vi "Display AppBar.vi"(8 "error in (no error)":errorcluster, 9 "AppBar Enqueuer":refnum<class "Message Enqueuer.lvclass">, 11 "MainController in":refnum<class "MainController.lvclass">) -> (0 "error out":errorcluster, 3 "MainController out":refnum<class "MainController.lvclass">)   [LabVIEW 2012, in "Win8uiFramework.lvlib" / "MainController.lvclass"]
uses:
  MainController.lvclass
  <vilib>/ActorFramework/Message Enqueuer/Message Enqueuer.lvclass
  Visibility Direction.ctl
  Visiblity States.ctl
  MainController.lvclass/MainController.ctl
  Insert Into SubPanel Msg.lvclass/Insert Into SubPanel Msg.ctl
  <vilib>/ActorFramework/Message Enqueuer/Message Enqueuer.lvclass/Message Enqueuer.ctl
  Read AppBar SubPanel.vi
  Read AppBar Enqueuer.vi
  Read AppBar State.vi
  Write AppBar Enqueuer.vi
  Write AppBar State.vi
  <vilib>/ActorFramework/Message Enqueuer/Enqueue.vi
  <vilib>/ActorFramework/Message Priority Queue/Priority Enqueue.vi
  <vilib>/Utility/error.llb/Simple Error Handler.vi
  Insert Into SubPanel Msg.lvclass
  Win8uiFramework.lvlib
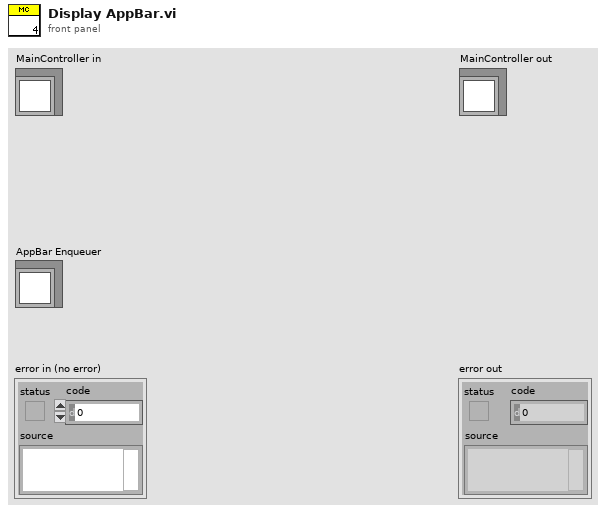
[diagram p1: front panel]
types:
  T1 = typedef "Win8uiFramework.lvlib/MainController.lvclass/Visiblity States.ctl" = enum16{"Disabled", "Hidden - Unpopulated", "Hidden - Populated", "Visible"}
  T2 = typedef "Win8uiFramework.lvlib/Visibility Direction.ctl" = enum16{"Show", "Hide"}
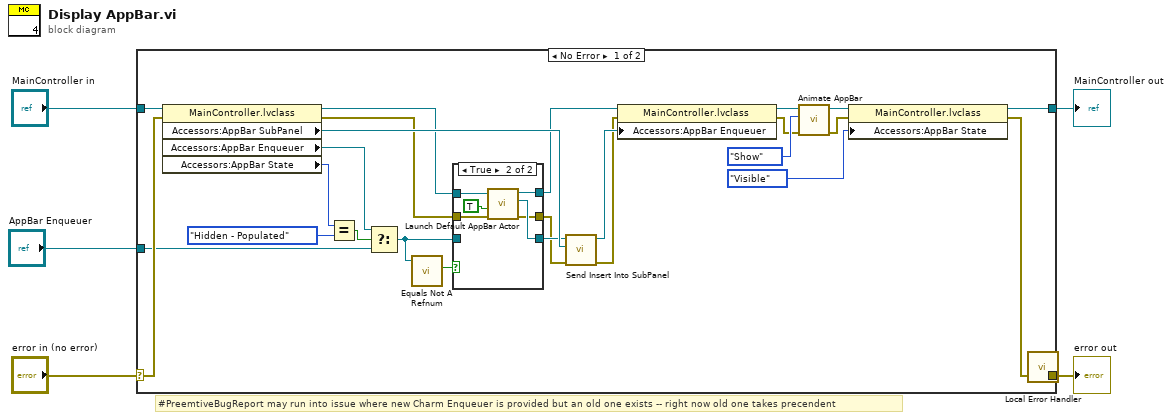
[diagram p0: block diagram]
diagram:
  # "#PreemtiveBugReport may run into issue where new Charm Enqueuer is provided but an old one exists -- right now old one takes precendent"
  n1 = case shown="No Error" "error in (no error)" {
    selector: "error in (no error)" -> [w26 w42]
    tunnel: [w6 w42] -> w4
    tunnel: [w22 w41] -> w2
    tunnel: "MainController in" -> [w31 w41]
    tunnel: "AppBar Enqueuer" -> [w18 _]
    frame No Error {
      n2 = property class="MainController.lvclass"(reference=w31, error in=w26) -> (reference out=w10:refnum<class "MainController.lvclass">, error out=w12:errorcluster, "Accessors:AppBar SubPanel"=w29:refnum<vi>, "Accessors:AppBar Enqueuer"=w15:refnum<class "Message Enqueuer.lvclass">, "Accessors:AppBar State"=w17:T1)
      n3 = Equal?(x=w17, y=Visiblity_States."Hidden - Populated") -> (x = y?=w19:bool)
      n4 = Select(t=w15, s=w19, f=w18) -> (s? t:f=w13:refnum<class "Message Enqueuer.lvclass">)
      n5 = call <vilib>:"Equals Not A Refnum.vi"("Message Enqueuer"=w13) -> ("Not a refnum?"=w14:bool)  [unwired: 10 in]
      n6 = case shown="True" w14 {
        tunnel: w13 -> [w34 _]
        tunnel: w10 -> [w33 w40]
        tunnel: w12 -> [w32 w39]
        tunnel: [w34 w38] -> w11
        tunnel: [w33 w37] -> w9
        tunnel: [w32 w36] -> w8
        frame False {
        }
        frame True {
          n7 = call-dynamic "Launch Default AppBar Actor.vi"("error in (no error)"=w39, "Stop Existing? (T)"=TRUE, "MainController in"=w40) -> ("error out"=w36:errorcluster, "Enqueuer"=w38:refnum<class "Message Enqueuer.lvclass">, "MainController out"=w37:refnum<class "MainController.lvclass">)  [unwired: 6 in]
        }
      }
      n8 = call "Send Insert Into SubPanel.vi"("error in (no error)"=w8, "SubPanel Ref"=w29, "Message Enqueuer"=w11) -> ("error out"=w25:errorcluster, "Message Enqueuer out"=w27:refnum<class "Message Enqueuer.lvclass">)  [unwired: 7 in]
      n9 = property class="MainController.lvclass"(reference=w9, error in=w25, "Accessors:AppBar Enqueuer"=w27) -> (reference out=w28:refnum<class "MainController.lvclass">, error out=w24:errorcluster)
      n10 = call-dynamic "Animate AppBar.vi"("error in (no error)"=w24, "Direction"=Visibility_Direction."Show", "MainController in"=w28) -> ("error out"=w21:errorcluster, "MainController out"=w23:refnum<class "MainController.lvclass">)  [unwired: 7 in]
      n11 = property class="MainController.lvclass"(reference=w23, error in=w21, "Accessors:AppBar State"=Visiblity_States."Visible" ("Charm State")) -> (reference out=w22:refnum<class "MainController.lvclass">, error out=w7:errorcluster)
      n12 = call "Local Error Handler.vi"("error in (no error)"=w7) -> ("error out"=w6:errorcluster)  [unwired: 18 in]
    }
    frame Error {
    }
  }
  "error out" <- w4
  "MainController out" <- w2
